vi "Peak Width.vi"(6 "Peak Y":dbl, 9 "Peak X":dbl, 10 "Y":dbl[](array[numeric]), 11 "X":dbl[](array[numeric])) -> (1 "low side":dbl, 2 "high side":dbl, 3 "width":dbl)   [LabVIEW 2016]
panel:
  out "Detected peak width":cluster{"X":dbl[], "Y":dbl[]}[](graph)
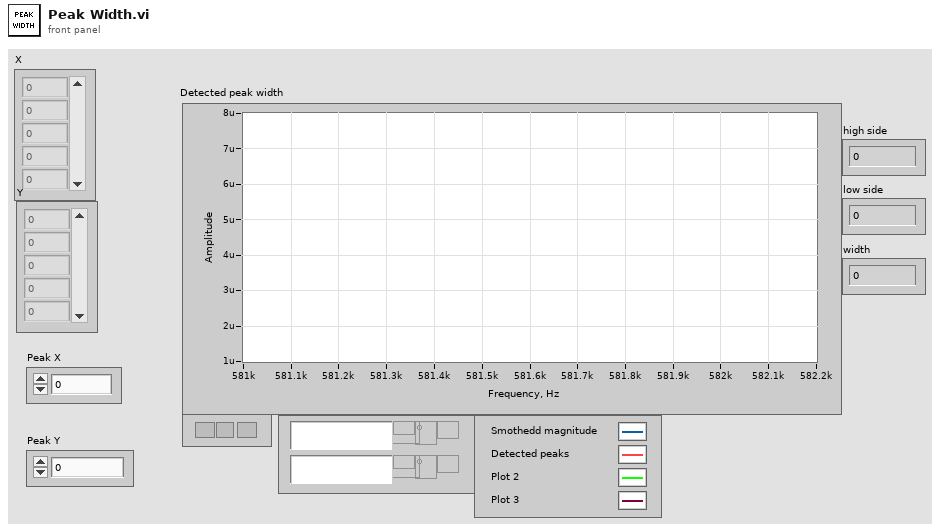
[diagram p1: front panel]
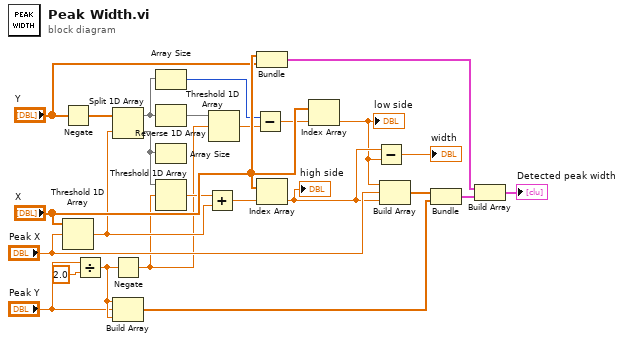
[diagram p0: block diagram]
diagram:
  n1 = Negate(x="Y") -> (-x=w7:dbl[])
  n2 = Threshold 1D Array(2:"Peak X", 3:"X") -> (0:w19:dbl)  [unwired: 1 in]
  n3 = Divide(x="Peak Y", y=2.0) -> (x/y=w17:dbl)
  n4 = Split 1D Array(array=w7, index=w19) -> (first subarray=w4:dbl[], second subarray=w21:dbl[])
  n5 = Negate(x=w17) -> (-x=w5:dbl)
  n6 = Build Array(w17, "Peak Y", w17) -> (w14:dbl[])
  n7 = Array Size(array=w4) -> (size(s)=w3:i32)
  n8 = Reverse 1D Array(array=w4) -> (reversed array=w6:dbl[])
  n9 = Array Size(array=w21) -> ()  [unwired: 1 out]
  n10 = Threshold 1D Array(2:w5, 3:w21) -> (0:w12:dbl)  [unwired: 1 in]
  n11 = Add(x=w12, y=w19) -> (x+y=w20:dbl)
  n12 = Threshold 1D Array(2:w5, 3:w6) -> (0:w2:dbl)  [unwired: 1 in]
  n13 = Subtract(x=w3, y=w2) -> (x-y=w1:dbl)
  n14 = Bundle("X"="X", "Y"="Y") -> (w25:cluster{"X":dbl[], "Y":dbl[]})  [unwired: 1 in]
  n15 = Index Array(array="X", index=w20) -> (element=w10:dbl)
  "high side" <- w10
  n16 = Index Array(array="X", index=w1) -> (element=w9:dbl)
  "low side" <- w9
  n17 = Subtract(x=w10, y=w9) -> (x-y=→"width":dbl)
  n18 = Build Array(w9, "Peak X", w10) -> (w15:dbl[])
  n19 = Bundle(w15, w14) -> (w13:cluster{dbl[], dbl[]})  [unwired: 1 in]
  n20 = Build Array(w25, w13) -> (→"Detected peak width":cluster{"X":dbl[], "Y":dbl[]}[])
